vi "get Columns and data.vi"(11 "数组":variant[](array[variant])) -> (2 "data":string[](array[string]), 3 "columns":string[](array[string]))   [LabVIEW 2016]
uses:
  <vilib>/addons/database/_DB Variant To Data/Database Variant To Data.xnode
  <vilib>/Utility/VariantDataType/VariantType.lvlib
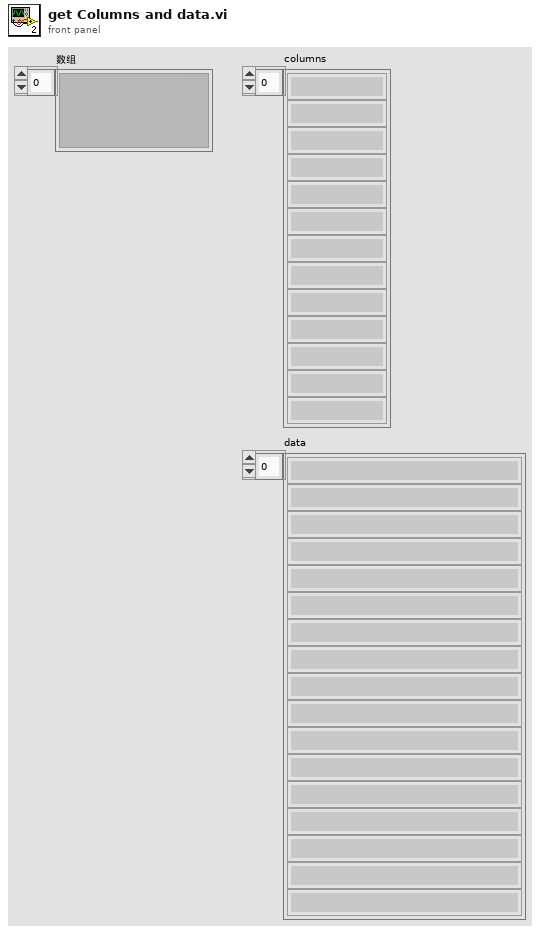
[diagram p1: front panel]
types:
  T1 = typedef "VariantType.lvlib/Type.ctl" = enum8{"Invalid Type", "Void", "I8", "I16", "I32", "I64", "U8", "U16", "U32", "U64", "Single Float", "Double Float", "Extended Float", "Single Complex", "Double Complex", "Extended Complex", "Enum U8", "Enum U16", "Enum U32", "Enum U64", "Single Float With Unit", "Double Float With Unit", "Extended Float With Unit", "Single Complex with Unit", "Double Complex with Unit", "Extended Complex with Unit", "Boolean", "String", "Path", "Picture", "Tag", "Array", "Cluster", "Variant", "LV Variant", "Waveform", "Timestamp", "Digital Waveform", "Digital Data", "ExpressData", "Refnum", "External Data", "VI", "Poly VI", "LabVIEW Class Instance", "Fixed Point"}
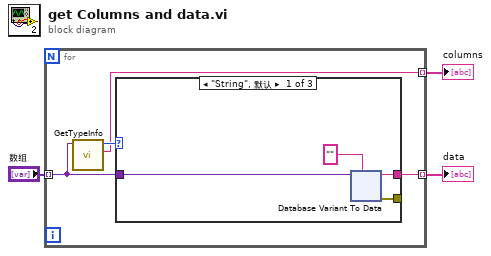
[diagram p0: block diagram]
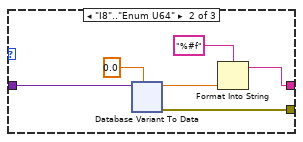
[diagram p2: hidden frame]
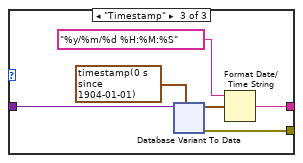
[diagram p3: hidden frame]
diagram:
  n1 = for {
    tunnel: [w7] -> w2 mode=indexing
    tunnel: "数组" -> [w5] mode=indexing
    tunnel: [w4] -> w3 mode=indexing
    n2 = call <vilib>:"GetTypeInfo.vi"("Variant"=w5) -> ("Name"=w4:string, "Type Enum"=w6:T1)  [unwired: 6 in, 3 out]
    n3 = case shown="\"String\", 默认" w6 {
      tunnel: [w9 w48 w84] -> w7
      tunnel: [w10 w49 w83] -> _
      tunnel: w5 -> [w8 w44 w82]
      frame "String", Default {
        n4 = xnode "Database Variant To Data"("database variant"=w8, "type"="") -> ("data"=w9:string, "error out"=w10:errorcluster)  [unwired: 1 in]
      }
      frame "I8".."Enum U64" {
        n5 = xnode "Database Variant To Data"("database variant"=w44, "type"=0.0) -> ("data"=w46:dbl, "error out"=w49:errorcluster)  [unwired: 1 in]
        n6 = Format Into String(format string="%#f" ("格式字符串"), w46) -> (resulting string=w48:string)  [unwired: 2 in, 1 out]
      }
      frame "Timestamp" {
        n7 = xnode "Database Variant To Data"("database variant"=w82, "type"=timestamp(0 s since 1904-01-01) ("当前时间")) -> ("data"=w87:timestamp, "error out"=w83:errorcluster)  [unwired: 1 in]
        n8 = Format Date/Time String(time format string (%c)="%y/%m/%d %H:%M:%S" ("时间格式字符串(%c)"), seconds (now)=w87) -> (date/time string=w84:string)  [unwired: 1 in]
      }
    }
  }
  "data" <- w2
  "columns" <- w3
